vi "ASI Positions and Console.vi"(0 "VISA in":refnum<visa-resource-name>, 1 "refresh rate [ms]":u32=250 min=50 step=10, 6 "Array of positions [internal units]":dbl[](array[numeric])=[0.0, 0.0, 0.0, 0.0, 0.0, 0.0, 0.0, 0.0, 0.0, 0.0] caption="Positions [mm]" step=100.0 format="%#_8f") -> (4 "VISA out":refnum<visa-resource-name>, 15 "error out":errorcluster)   [LabVIEW 2014]
doc: "Top-level VI for continuously querying the position of the specified axes."
uses:
  <instrlib>/ASI TG-1000/Public/Utility/Axis Name.ctl
  <instrlib>/ASI TG-1000/ASI TG-1000.lvlib
panel:
  out "error out update loop":errorcluster
  out "error out event loop":errorcluster
  in  "Move home":bool
  out "Array of status strings":string[](array[string]) caption="Status strings"
  out "Serial response":string
  in  "Send serial command":bool
  in  "Serial command string":string
  in  "Halt movement":bool
  in  "Position step":dbl=100.0
  out "Motors Busy?":bool
  in  "Save Position to File":bool
  in  "Set Position from file":bool
  in  "file path":path
  in  "Array of axes":T1[](array[typedef])=[enum."X", enum."Y", enum."Z", enum."F", enum."P", enum."Q", enum."A", enum."B", enum."C", enum."D"]
  in  "Stop program":bool
  # "the stages positions unit   is mm and the internal unit is 0.1um by default"
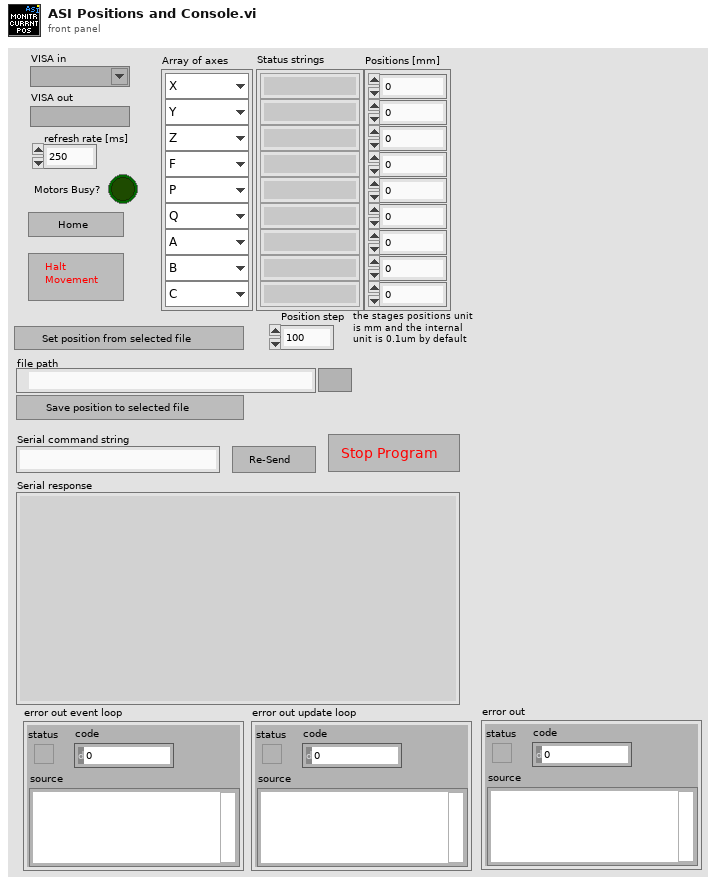
[diagram p1: front panel]
types:
  T1 = typedef "ASI TG-1000.lvlib/Axis Name.ctl" = enum8{"undefined", "A", "B", "C", "D", "E", "F", "G", "H", "I", "J", "K", "L", "M", "N", "O", "P", "Q", "R", "S", "T", "U", "V", "W", "X", "Y", "Z"}
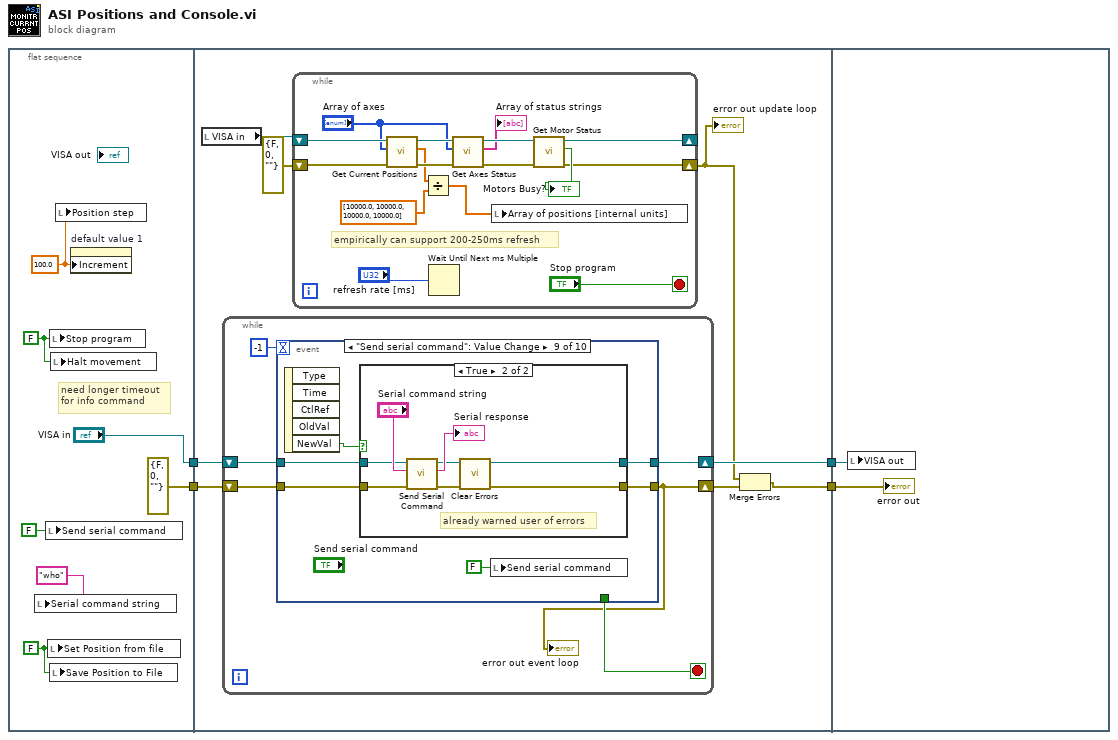
[diagram p0: block diagram]
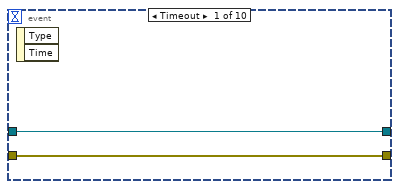
[diagram p2: hidden frame]
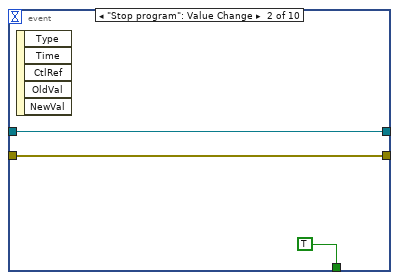
[diagram p3: hidden frame]
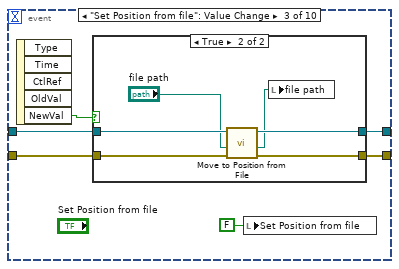
[diagram p4: hidden frame]
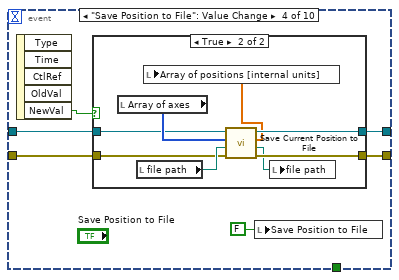
[diagram p6: hidden frame]
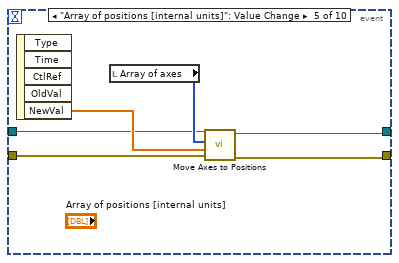
[diagram p8: hidden frame]
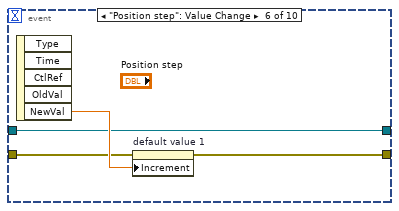
[diagram p9: hidden frame]
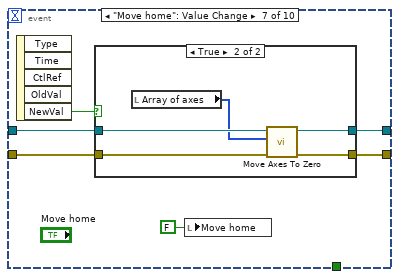
[diagram p10: hidden frame]
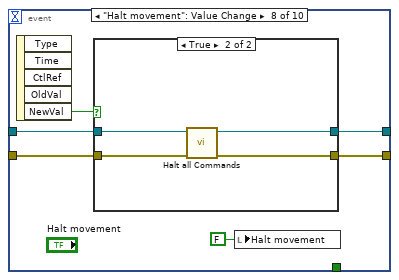
[diagram p12: hidden frame]
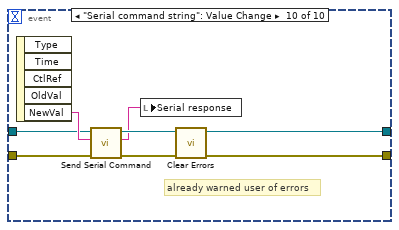
[diagram p15: hidden frame]
diagram:
  n1 = flat-sequence {
    tunnel: [errorcluster {"status"=FALSE, "code"=0, "source"=""} ("error out")] -> w2
    tunnel: ["VISA in"] -> w1
    tunnel: [w19] -> w4
    tunnel: [w14] -> w3
    tunnel: w2 -> [w17]
    tunnel: w1 -> [w18]
    tunnel: w4 -> [w134]
    tunnel: w3 -> [w135]
    frame #0 {
      w9 = FALSE ("Set Position from file")
      w7 = 100.0 ("Position inc/dec step")
      w8 = FALSE ("stop")
      # "need longer timeout\nfor info command"
      n2 = local write "Serial command string"("who" ("Serial command string")) -> ()
      n3 = local write "Send serial command"(FALSE ("Send serial command")) -> ()
      n4 = local write "Set Position from file"(w9) -> ()
      n5 = local write "Stop program"(w8) -> ()
      n6 = local write "Save Position to File"(w9) -> ()
      n7 = local write "Halt movement"(w8) -> ()
      n8 = local write "Position step"(w7) -> ()
      n9 = property on="default value 1" class="DigNum (strict)"("Increment"=w7) -> ()  [unwired: 2 in, 2 out]
    }
    frame #1 {
      n10 = local read "VISA in"() -> (w16:refnum<visa-resource-name>)
      n11 = while {
        shift-right: [w40] -> w13
        shift-left: w17 -> [w39]
        shift-right: [w37] -> w19
        shift-left: w18 -> [w38]
        stop <- w41 stop-if-true
        n12 = event shown="[8] \"Send serial command\": Value Change" {
          selector: _ -> [_ _ _ _ _ _ _ _ _ _]
          dyn-events: _ -> [_ _ _ _ _ _ _ _ _ _]
          timeout: -1 -> [_ _ _ _ _ _ _ _ _ _]
          tunnel: [_ TRUE _ _ _ _ _ _ _ _] -> w41
          tunnel: [w43 w45 w50 w63 w80 w84 w87 w102 w114 w127] -> w40
          tunnel: w39 -> [w43 w45 w49 w64 w79 w85 w90 w103 w115 w130]
          tunnel: w38 -> [w42 w44 w48 w62 w78 w83 w89 w101 w113 w132]
          tunnel: [w42 w44 w47 w61 w77 w83 w88 w100 w112 w131] -> w37
          event Timeout {
            n13 = event-data() -> ()  [unwired: 1 in, 2 out]
          }
          event "Stop program": Value Change {
            n14 = event-data() -> ()  [unwired: 1 in, 5 out]
          }
          event "Set Position from file": Value Change {
            n15 = event-data() -> ("NewVal"=w52:bool)  [unwired: 1 in, 4 out]
            n16 = case shown="True" w52 {
              tunnel: [w54 w60] -> w50
              tunnel: w49 -> [w54 w59]
              tunnel: w48 -> [w53 w58]
              tunnel: [w53 w57] -> w47
              frame False {
              }
              frame True {
                n17 = call <instrlib>:"Move to Position from File.vi"("error in (no error)"=w59, "file path in"="file path", "VISA in"=w58) -> ("error out"=w60:errorcluster, "file path out"=w56:path, "VISA out"=w57:refnum<visa-resource-name>)  [unwired: 6 in]
                n18 = local write "file path"(w56) -> ()
              }
            }
            n19 = local write "Set Position from file"(FALSE ("Set Position from file")) -> ()
          }
          event "Save Position to File": Value Change {
            n20 = event-data() -> ("NewVal"=w66:bool)  [unwired: 1 in, 4 out]
            n21 = case shown="True" w66 {
              tunnel: w64 -> [w68 w74]
              tunnel: [w68 w73] -> w63
              tunnel: w62 -> [w67 w72]
              tunnel: [w67 w71] -> w61
              frame False {
              }
              frame True {
                n22 = local read "Array of axes"() -> (w75:T1[])
                n23 = local read "file path"() -> (w76:path)
                n24 = call <instrlib>:"Save Current Position to File.vi"("error in (no error)"=w74, "file path"=w76, "Array of axes"=w75, "VISA in"=w72) -> ("error out"=w73:errorcluster, "file path out"=w70:path, "Array of positions [um]"=w69:dbl[], "VISA out"=w71:refnum<visa-resource-name>)  [unwired: 4 in]
                n25 = local write "Array of positions [internal units]"(w69) -> ()
                n26 = local write "file path"(w70) -> ()
              }
            }
            n27 = local write "Save Position to File"(FALSE ("Save Position to File")) -> ()
          }
          event "Array of positions [internal units]": Value Change {
            n28 = event-data() -> ("NewVal"=w82:dbl[])  [unwired: 1 in, 4 out]
            n29 = local read "Array of axes"() -> (w81:T1[])
            n30 = call <instrlib>:"Move Axes to Positions.vi"("error in (no error)"=w79, "Array of positions [internal units]"=w82, "Array of axes"=w81, "VISA in"=w78) -> ("error out"=w80:errorcluster, "VISA out"=w77:refnum<visa-resource-name>)  [unwired: 5 in]
          }
          event "Position step": Value Change {
            n31 = event-data() -> ("NewVal"=w86:dbl)  [unwired: 1 in, 4 out]
            n32 = property on="default value 1" class="DigNum (strict)"(error in=w85, "Increment"=w86) -> (error out=w84:errorcluster)  [unwired: 1 in, 1 out]
          }
          event "Move home": Value Change {
            n33 = event-data() -> ("NewVal"=w92:bool)  [unwired: 1 in, 4 out]
            n34 = case shown="True" w92 {
              tunnel: w90 -> [w93 w96]
              tunnel: w89 -> [w94 w99]
              tunnel: [w94 w98] -> w88
              tunnel: [w93 w97] -> w87
              frame False {
              }
              frame True {
                n35 = local read "Array of axes"() -> (w95:T1[])
                n36 = call <instrlib>:"Move Axes To Zero.vi"("error in (no error)"=w96, "Array of axes"=w95, "VISA in"=w99) -> ("error out"=w97:errorcluster, "VISA out"=w98:refnum<visa-resource-name>)  [unwired: 6 in]
              }
            }
            n37 = local write "Move home"(FALSE ("Move home")) -> ()
          }
          event "Halt movement": Value Change {
            n38 = event-data() -> ("NewVal"=w105:bool)  [unwired: 1 in, 4 out]
            n39 = case shown="True" w105 {
              tunnel: w103 -> [w107 w111]
              tunnel: [w107 w110] -> w102
              tunnel: w101 -> [w106 w109]
              tunnel: [w106 w108] -> w100
              frame False {
              }
              frame True {
                n40 = call <instrlib>:"Halt all Commands.vi"("error in (no error)"=w111, "VISA in"=w109) -> ("error out"=w110:errorcluster, "VISA out"=w108:refnum<visa-resource-name>)  [unwired: 7 in]
              }
            }
            n41 = local write "Halt movement"(FALSE ("Halt movement")) -> ()
          }
          event "Send serial command": Value Change {
            n42 = event-data() -> ("NewVal"=w116:bool)  [unwired: 1 in, 4 out]
            n43 = case shown="True" w116 {
              tunnel: w115 -> [w119 w125]
              tunnel: [w119 w120] -> w114
              tunnel: w113 -> [w118 w122]
              tunnel: [w118 w121] -> w112
              frame False {
              }
              frame True {
                # "already warned user of errors"
                n44 = call <instrlib>:"Send Serial Command.vi"("error in (no error)"=w125, "Command"="Serial command string", "VISA in"=w122) -> ("error out"=w124:errorcluster, "Response"=→"Serial response":string, "VISA out"=w121:refnum<visa-resource-name>)  [unwired: 6 in]
                n45 = call <vilib>:"Clear Errors.vi"("error in (no error)"=w124) -> ("error out"=w120:errorcluster)  [unwired: 5 in, 1 out]
              }
            }
            n46 = local write "Send serial command"(FALSE ("Send serial command")) -> ()
          }
          event "Serial command string": Value Change {
            # "already warned user of errors"
            n47 = event-data() -> ("NewVal"=w133:string)  [unwired: 1 in, 4 out]
            n48 = call <instrlib>:"Send Serial Command.vi"("error in (no error)"=w130, "Command"=w133, "VISA in"=w132) -> ("error out"=w129:errorcluster, "Response"=w128:string, "VISA out"=w131:refnum<visa-resource-name>)  [unwired: 6 in]
            n49 = local write "Serial response"(w128) -> ()
            n50 = call <vilib>:"Clear Errors.vi"("error in (no error)"=w129) -> ("error out"=w127:errorcluster)  [unwired: 5 in, 1 out]
          }
        }
        "error out event loop" <- w40
      }
      n51 = while {
        shift-right: [w25] -> _
        shift-left: w16 -> [w27]
        shift-right: [w24] -> w12
        shift-left: errorcluster {"status"=FALSE, "code"=0, "source"=""} ("error out") -> [w26]
        stop <- "Stop program" stop-if-true
        # "empirically can support 200-250ms refresh"
        n52 = call <instrlib>:"Get Current Positions.vi"("error in (no error)"=w26, "Array of axes"="Array of axes", "VISA in"=w27) -> ("error out"=w33:errorcluster, "Array of positions [internal units]"=w22:dbl[], "VISA out"=w34:refnum<visa-resource-name>)  [unwired: 6 in]
        n53 = Divide(x=w22, y=dbl[] [10000.0, 10000.0, 10000.0, 10000.0]) -> (x/y=w20:dbl[])
        n54 = Wait Until Next ms Multiple(millisecond multiple="refresh rate [ms]") -> ()  [unwired: 1 out]
        n55 = call <instrlib>:"Get Axes Status.vi"("error in (no error)"=w33, "Array of axes"="Array of axes", "VISA in"=w34) -> ("error out"=w32:errorcluster, "Array of status strings"=→"Array of status strings":string[], "VISA out"=w31:refnum<visa-resource-name>)  [unwired: 6 in]
        n56 = local write "Array of positions [internal units]"(w20) -> ()
        n57 = call <instrlib>:"Get Motor Status.vi"("error in (no error)"=w32, "VISA in"=w31) -> ("error out"=w24:errorcluster, "Motors Busy?"=→"Motors Busy?":bool, "VISA out"=w25:refnum<visa-resource-name>)  [unwired: 6 in]
      }
      "error out update loop" <- w12
      n58 = Merge Errors(w12, w13) -> (w14:errorcluster)
    }
    frame #2 {
      n59 = local write "VISA out"(w134) -> ()
      "error out" <- w135
    }
  }
